vi "Set_PointListBox.vi"(11 "Table":string[][](array[string])) -> (3 "Point":string[](array[string]))   [LabVIEW 2019]
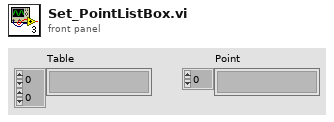
[diagram p1: front panel]
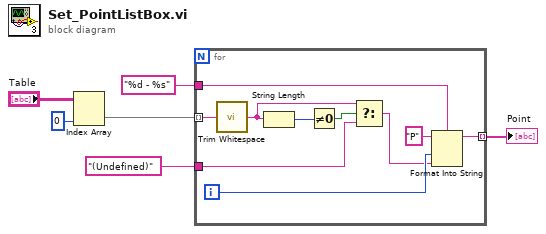
[diagram p0: block diagram]
diagram:
  n1 = Index Array(array="Table", index (col)=0 ("disabled index (col)")) -> (element=w3:string[])  [unwired: 1 in]
  n2 = for {
    tunnel: w3 -> [w16] mode=indexing
    tunnel: [w9] -> w4 mode=indexing
    tunnel: "(Undefined)" ("f") -> [w8]
    tunnel: "%d - %s" ("format string") -> [w7]
    i -> [w11]
    n3 = call <vilib>:"Trim Whitespace.vi"("string"=w16) -> ("trimmed string"=w13:string)  [unwired: 1 in]
    n4 = String Length(string=w13) -> (length=w15:i32)
    n5 = Not Equal To 0?(x=w15) -> (x != 0?=w14:bool)
    n6 = Select(t=w13, s=w14, f=w8) -> (s? t:f=w10:string)
    n7 = Format Into String(format string=w7, initial string="P", w11, w10) -> (resulting string=w9:string)  [unwired: 1 in, 1 out]
  }
  "Point" <- w4
